vi "Theme4_Topic4_qn23.vi"(9 "RefPrevious":refnum<vi>, 10 "RefNext":refnum<vi>, 11 "connection reference":T1) -> (2 "AnsIndicator":refnum<vi>[](array[refnum]))   [LabVIEW 2013]
uses:
  why.vi
  Precontrol.vi
  <vilib>/addons/database/Connection.llb/Conn ObjectReference.ctl
  <vilib>/addons/database/NI_Database_API.lvlib
panel:
  out "Why?":string
  out "DInd":bool
  out "CInd":bool
  out "BInd":bool
  out "AInd":bool
  in  "ABCD":enum32{"No Selection", "A", "B", "C", "D"}(radio)
  out "MCQ_Randomized":string[](array[string])
  # "A cow heard something that the farmer could net hear . Given that the wavelength of the sound heard by the cow is 1.0 cm, which of the following is a possible audible fvrequency range of the cow?"
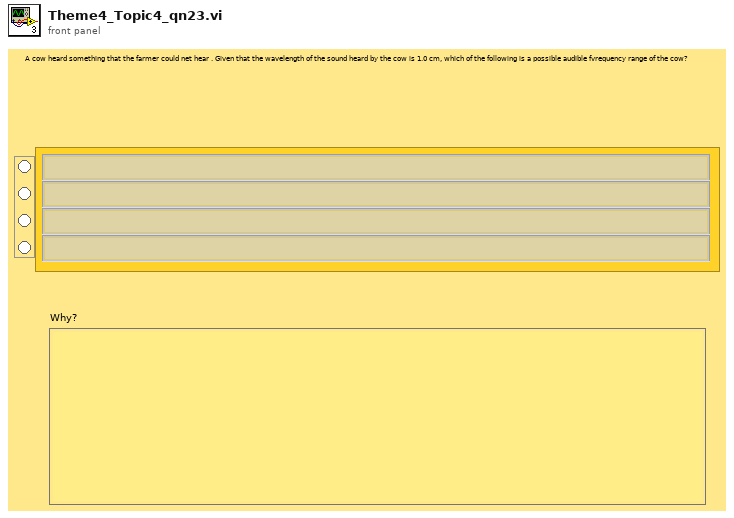
[diagram p1: front panel]
types:
  T1 = typedef "NI_Database_API.lvlib/Conn ObjectReference.ctl" = refnum<k1>
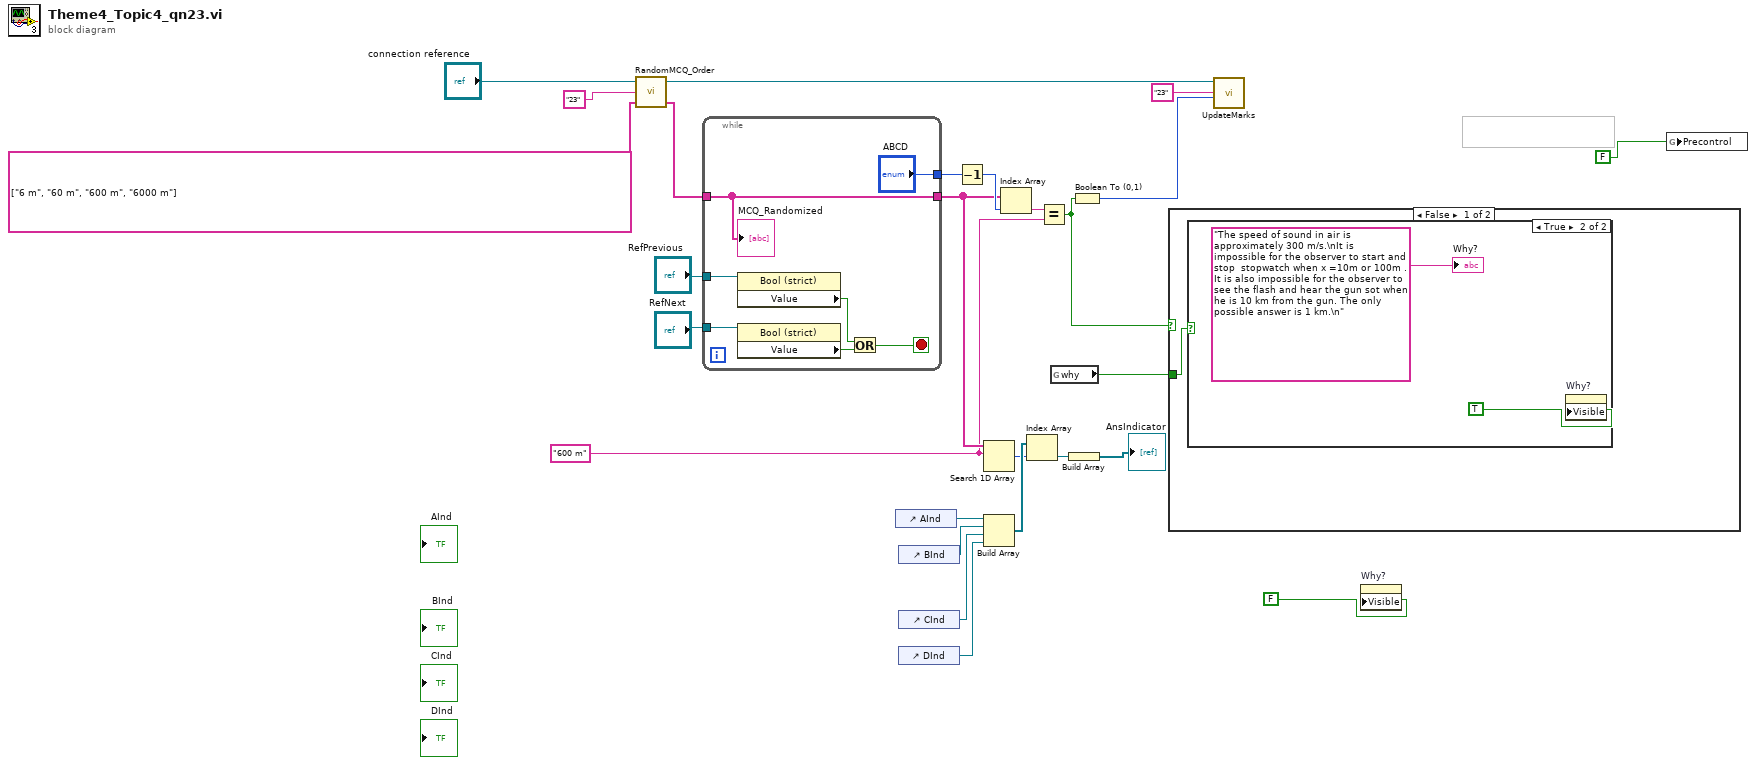
[diagram p0: block diagram]
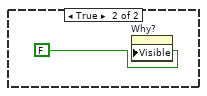
[diagram p3: hidden frame]
diagram:
  w13 = "600 m" ("element")
  n1 = call "RandomMCQ_Order.vi"("MCQ_Ordered"=string[] ["6 m", "60 m", "600 m", "6000 m"], "Questions_Ordered"="23", "connection reference"="connection reference") -> ("MCQ_Randomized"=w26:string[], "connection reference out"=w10:T1)  [unwired: 1 in]
  n2 = while {
    tunnel: ["ABCD"] -> w2
    tunnel: w26 -> [w28]
    tunnel: [w28] -> w15
    tunnel: "RefNext" -> [w29]
    tunnel: "RefPrevious" -> [w30]
    stop <- w27 stop-if-true
    n3 = property class="Bool (strict)"(reference=w30) -> ("Value"=w32:bool)  [unwired: 1 in, 2 out]
    n4 = property class="Bool (strict)"(reference=w29) -> ("Value"=w31:bool)  [unwired: 1 in, 2 out]
    n5 = Or(x=w32, y=w31) -> (x .or. y?=w27:bool)
    "MCQ_Randomized" <- w28
  }
  n6 = control-ref of="AInd"() -> (w23:refnum<vi>)
  n7 = control-ref of="BInd"() -> (w22:refnum<vi>)
  n8 = control-ref of="CInd"() -> (w21:refnum<vi>)
  n9 = control-ref of="DInd"() -> (w20:refnum<vi>)
  n10 = Decrement(x=w2) -> (x-1=w16:enum32{"No Selection", "A", "B", "C", "D"})
  n11 = Search 1D Array(1D array=w15, element=w13) -> (index of element=w18:i32)  [unwired: 1 in]
  n12 = Build Array(w23, w22, w21, w20) -> (w19:refnum<vi>[])
  n13 = Index Array(array=w15, index=w16) -> (element=w14:string)
  n14 = Index Array(array=w19, index=w18) -> (element=w17:refnum<vi>)
  n15 = Equal?(x=w14, y=w13) -> (x = y?=w5:bool)
  n16 = global read "why.vi" "why"() -> (w3:bool)
  n17 = Build Array(w17) -> (→"AnsIndicator":refnum<vi>[])
  n18 = Boolean To (0,1)(Boolean=w5) -> (0, 1=w6:i16)
  n19 = case shown="False" w5 {
    tunnel: w3 -> [w34 _]
    frame False {
      n20 = case shown="True" w34 {
        frame False {
        }
        frame True {
          n21 = property on="Why?" class="Str"("Visible"=TRUE) -> ()  [unwired: 2 in, 2 out]
          "Why?" <- "The speed of sound in air is approximately 300 m/s.\nIt is impossible for the observer to start and stop  stopwatch when x =10m or 100m . It is also impossible for the observer to see the flash and hear the gun sot when he is 10 km from the gun. The only possible answer is 1 km.\n"
        }
      }
    }
    frame True {
      n22 = property on="Why?" class="Str"("Visible"=FALSE) -> ()  [unwired: 2 in, 2 out]
    }
  }
  n23 = call "UpdateMarks.vi"("MarksEarned"=w6, "QuestionsNo_Ordered"="23", "connection reference"=w10) -> ()  [unwired: 9 in]
  n24 = property on="Why?" class="Str"("Visible"=FALSE) -> ()  [unwired: 2 in, 2 out]
  n25 = global write "Precontrol.vi" "Precontrol"(FALSE) -> ()
